vi "Setup.vi"(10 "Attributes":refnum<class "Attributes.lvclass">, 11 "TEMPLATE Actor in":refnum<class "TEMPLATE Actor.lvclass">) -> (0 "Error out":errorcluster, 3 "TEMPLATE Actor out":refnum<class "TEMPLATE Actor.lvclass">)   [LabVIEW 2025, in "_Template.lvlib" / "Templates.lvlib" / "TEMPLATE Actor.lvlib" / "TEMPLATE Actor.lvclass"]
uses:
  TEMPLATE Actor.lvclass
  jettl/jettl/Attributes/Attributes/Attributes.lvclass
  jettl/jettl/Actor/Actor.lvclass
  TEMPLATE Actor.lvclass/TEMPLATE Actor.ctl
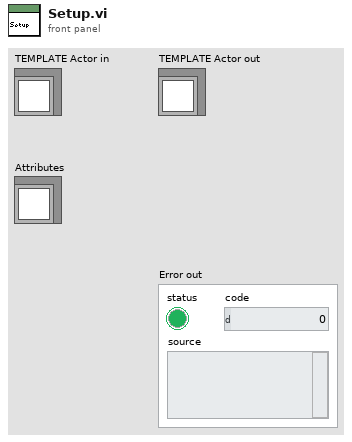
[diagram p1: front panel]
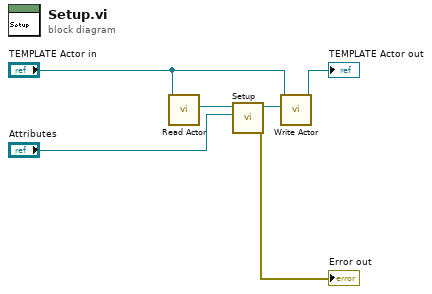
[diagram p0: block diagram]
diagram:
  n1 = call-dynamic "Read Actor.vi"("TEMPLATE Actor in"="TEMPLATE Actor in") -> ("Actor"=w2:refnum<class "Actor.lvclass">)  [unwired: 10 in]
  n2 = call-dynamic "Setup.vi"("Attributes"="Attributes", "Actor in"=w2) -> ("Error out"=→"Error out":errorcluster, "Actor out"=w3:refnum<class "Actor.lvclass">)  [unwired: 8 in]
  n3 = call-dynamic "Write Actor.vi"("Actor"=w3, "TEMPLATE Actor in"="TEMPLATE Actor in") -> ("TEMPLATE Actor out"=→"TEMPLATE Actor out":refnum<class "TEMPLATE Actor.lvclass">)  [unwired: 9 in]
